vi "NML_DATA_ACQ_Query_mem.vi"(2 "Enum":T1(ring)) -> (0 "error out 2":errorcluster, 1 "Value":variant)   [LabVIEW 2025]
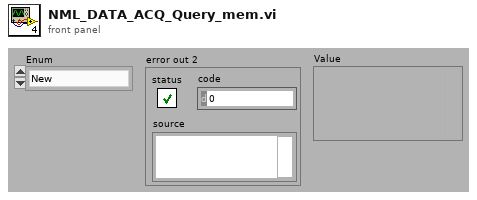
[diagram p1: front panel]
types:
  T1 = enum32{"New", "Trigger", "Delta Trigger", "Run", "comments"}
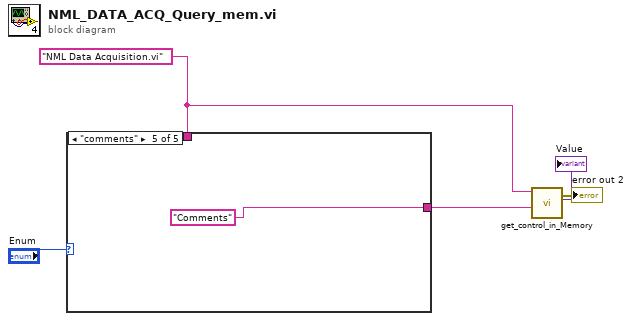
[diagram p0: block diagram]
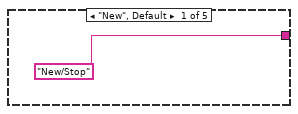
[diagram p2: hidden frame]
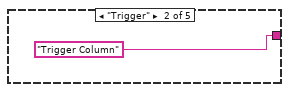
[diagram p3: hidden frame]
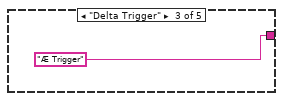
[diagram p4: hidden frame]
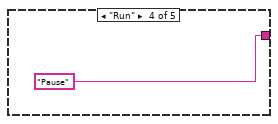
[diagram p5: hidden frame]
diagram:
  w4 = "NML Data Acquisition.vi" ("VI Name")
  n1 = case shown="\"comments\"" "Enum" {
    tunnel: w4 -> [_ _ _ _ _]
    tunnel: ["New/Stop" ("Control Name") "Trigger Column" ("Control Name") "Æ Trigger" ("Control Name") "Pause" ("Control Name") "Comments" ("Control Name")] -> w3
    frame "New", Default {
    }
    frame "Trigger" {
    }
    frame "Delta Trigger" {
    }
    frame "Run" {
    }
    frame "comments" {
    }
  }
  n2 = call "get_control_in_Memory.vi"("Control Name"=w3, "VI Name"=w4) -> ("error out 2"=→"error out 2":errorcluster, "Value"=→"Value":variant)  [unwired: 2 in]
